vi "Mapping Error Dialog (Multiple).vi"(8 "error in (no error)":errorcluster, 11 "Mapping Types":T2) -> (0 "error out":errorcluster, 3 "Continue?":bool)   [LabVIEW 2016, in "System Mapping Tool.lvlib"]
uses:
  System Mapping Tool.lvlib
  TypeDefs/Mapping Error Groups.ctl
panel:
  in  "Tab Control":T1(tab)
  in  "Mapping Errors":i32(listbox)
  in  "Existing Mappings":i32(listbox)
  in  "Imported Mappings":i32(listbox)
  in  "Continue":bool
  in  "Cancel":bool
  # "The following mappings will not be imported due to the designated error:"
  # "The following mappings will not be imported because they already exist in the system definition:"
  # "The following mappings will be imported:"
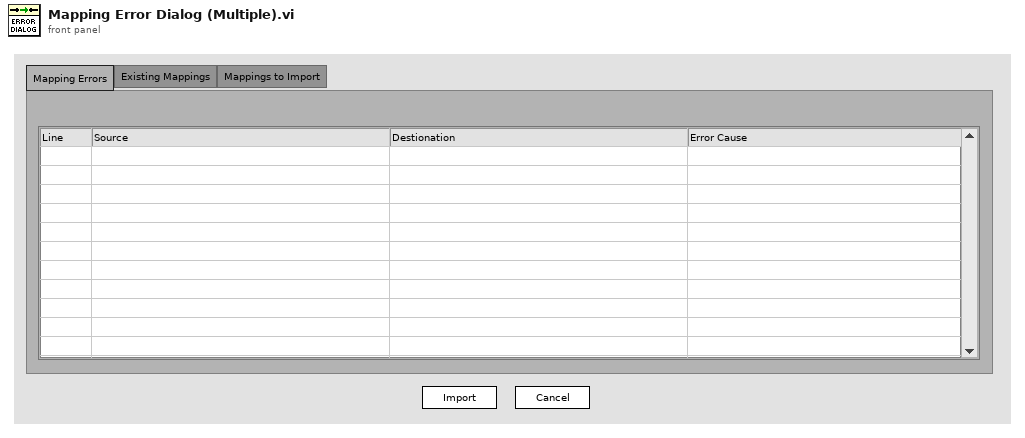
[diagram p1: front panel]
types:
  T1 = enum32{"Mapping Errors", "Existing Mappings", "Mappings to Import"}
  T2 = typedef "System Mapping Tool.lvlib/Mapping Error Groups.ctl" = cluster{"Mapping Errors":string[][], "Duplicate Mappings":string[][], "Mappings to Import":string[][]}
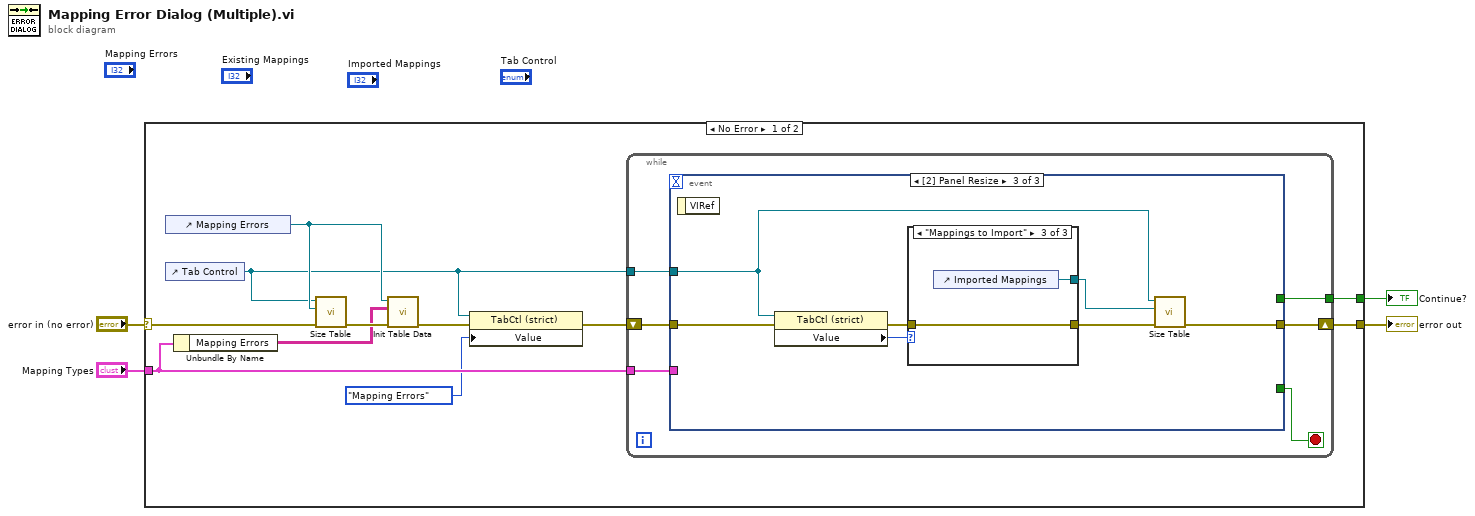
[diagram p0: block diagram]
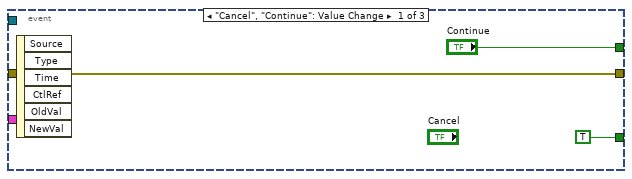
[diagram p2: hidden frame]
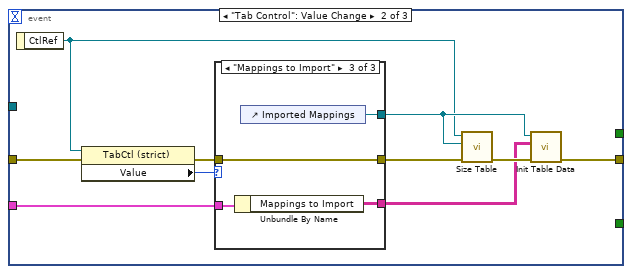
[diagram p3: hidden frame]
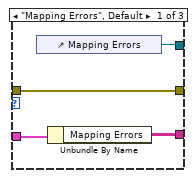
[diagram p4: hidden frame]
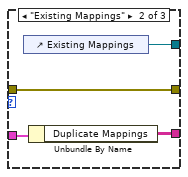
[diagram p5: hidden frame]
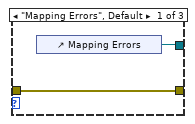
[diagram p6: hidden frame]
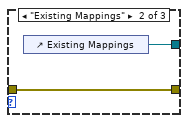
[diagram p7: hidden frame]
diagram:
  n1 = case shown="No Error" "error in (no error)" {
    selector: "error in (no error)" -> [w13 w60]
    tunnel: [w15 w60] -> w3
    tunnel: [w14 _] -> w2
    tunnel: "Mapping Types" -> [w8 _]
    frame No Error {
      n2 = control-ref of="Mapping Errors"() -> (w10:refnum<vi>)
      n3 = control-ref of="Tab Control"() -> (w6:refnum<vi>)
      n4 = Unbundle By Name(w8) -> ("Mapping Errors"=w9:string[][])
      n5 = call "Size Table.vi"("error in (no error)"=w13, "Table"=w10, "Tab Control"=w6) -> ("error out"=w12:errorcluster)  [unwired: 8 in]
      n6 = call "Init Table Data.vi"("error in (no error)"=w12, "Item Names"=w9, "Table"=w10) -> ("error out"=w11:errorcluster)  [unwired: 8 in]
      n7 = property class="TabCtl (strict)"(reference=w6, error in=w11, "Value"=T1."Mapping Errors") -> (error out=w7:errorcluster)  [unwired: 1 out]
      n8 = while {
        shift-right: [w20] -> w15
        shift-left: w7 -> [w21]
        tunnel: [w18] -> w14
        tunnel: w8 -> [w17]
        tunnel: w6 -> [w16]
        stop <- w19 stop-if-true
        n9 = event shown="[2] Panel Resize" {
          selector: _ -> [_ _ _]
          dyn-events: _ -> [_ _ _]
          timeout: _ -> [_ _ _]
          tunnel: w21 -> [w24 w34 w53]
          tunnel: [w24 w28 w49] -> w20
          tunnel: [TRUE _ _] -> w19
          tunnel: ["Continue" _ _] -> w18
          tunnel: w17 -> [_ w26 _]
          tunnel: w16 -> [_ _ w47]
          event "Cancel", "Continue": Value Change {
            n10 = event-data() -> ()  [unwired: 1 in, 6 out]
          }
          event "Tab Control": Value Change {
            n11 = event-data() -> ("CtlRef"=w27:refnum<vi>)  [unwired: 1 in]
            n12 = property class="TabCtl (strict)"(reference=w27, error in=w34) -> (error out=w32:errorcluster, "Value"=w33:T1)  [unwired: 1 out]
            n13 = case shown="\"Mappings to Import\"" w33 {
              tunnel: w32 -> [w37 w41 w45]
              tunnel: [w38 w42 w46] -> w30
              tunnel: [w37 w41 w45] -> w31
              tunnel: w26 -> [w36 w40 w44]
              tunnel: [w35 w39 w43] -> w25
              frame "Mapping Errors", Default {
                n14 = control-ref of="Mapping Errors"() -> (w38:refnum<vi>)
                n15 = Unbundle By Name(w36) -> ("Mapping Errors"=w35:string[][])
              }
              frame "Existing Mappings" {
                n16 = control-ref of="Existing Mappings"() -> (w42:refnum<vi>)
                n17 = Unbundle By Name(w40) -> ("Duplicate Mappings"=w39:string[][])
              }
              frame "Mappings to Import" {
                n18 = Unbundle By Name(w44) -> ("Mappings to Import"=w43:string[][])
                n19 = control-ref of="Imported Mappings"() -> (w46:refnum<vi>)
              }
            }
            n20 = call "Size Table.vi"("error in (no error)"=w31, "Table"=w30, "Tab Control"=w27) -> ("error out"=w29:errorcluster)  [unwired: 8 in]
            n21 = call "Init Table Data.vi"("error in (no error)"=w29, "Item Names"=w25, "Table"=w30) -> ("error out"=w28:errorcluster)  [unwired: 8 in]
          }
          event Panel Resize {
            n22 = event-data() -> ()  [unwired: 1 in, 1 out]
            n23 = property class="TabCtl (strict)"(reference=w47, error in=w53) -> (error out=w52:errorcluster, "Value"=w48:T1)  [unwired: 1 out]
            n24 = case shown="\"Mappings to Import\"" w48 {
              tunnel: w52 -> [w54 w56 w58]
              tunnel: [w55 w57 w59] -> w50
              tunnel: [w54 w56 w58] -> w51
              frame "Mapping Errors", Default {
                n25 = control-ref of="Mapping Errors"() -> (w55:refnum<vi>)
              }
              frame "Existing Mappings" {
                n26 = control-ref of="Existing Mappings"() -> (w57:refnum<vi>)
              }
              frame "Mappings to Import" {
                n27 = control-ref of="Imported Mappings"() -> (w59:refnum<vi>)
              }
            }
            n28 = call "Size Table.vi"("error in (no error)"=w51, "Table"=w50, "Tab Control"=w47) -> ("error out"=w49:errorcluster)  [unwired: 8 in]
          }
        }
      }
    }
    frame Error {
    }
  }
  "error out" <- w3
  "Continue?" <- w2
